vi "Create User Event - ExitEventLoop.vi"(8 "error in (no error)":errorcluster) -> (0 "error out":errorcluster, 2 "user event ExitEventLoop":refnum<user-event>, 3 "Event Registration Refnum":refnum<event-registration>)   [LabVIEW 2017, in "UserEvent-ExitEventLoop.lvlib"]
doc: "Create a boolean user event that will be used to stop the event loop from the message handling loop.\n\nBolder Software LLC"
uses:
  UserEvent-ExitEventLoop.lvlib
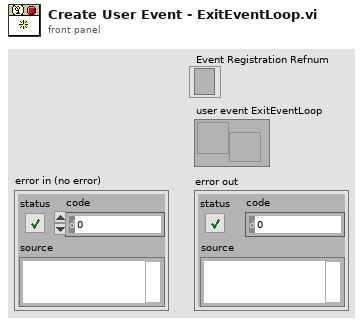
[diagram p1: front panel]
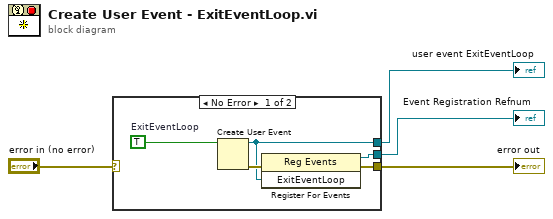
[diagram p0: block diagram]
diagram:
  n1 = case shown="No Error" "error in (no error)" {
    selector: "error in (no error)" -> [_ w10]
    tunnel: [w7 _] -> w4
    tunnel: [w6 _] -> w3
    tunnel: [w5 w10] -> w2
    frame No Error {
      w8 = TRUE  # ExitEventLoop
      n2 = Create User Event(user event datatype=w8) -> (user event=w7:refnum<user-event>, error out=w9:errorcluster)  [unwired: 1 in]
      n3 = register-events(error in=w9, w7) -> (reference out=w6:refnum<event-registration>, error out=w5:errorcluster)  [unwired: 1 in]
    }
    frame Error {
    }
  }
  "Event Registration Refnum" <- w3
  "user event ExitEventLoop" <- w4
  "error out" <- w2
